vi "GlobalIniInputOutput.vi"(9 "Read or Write":T1=enum."Read Key", 11 "Ini File Refnum":T2) -> ()   [LabVIEW 2014]
uses:
  <vilib>/Utility/config.llb/Config Data RefNum.ctl
  ReadWriteIniKey.ctl
  Robot Global Data.vi
  AutonCals.vi
  DriveCals.vi
  <vilib>/Utility/config.llb/NI_LVConfig.lvlib
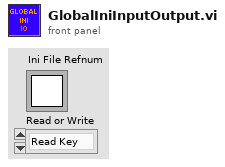
[diagram p1: front panel]
types:
  T1 = typedef "ReadWriteIniKey.ctl" = enum16{"Write Key", "Read Key"}
  T2 = typedef "NI_LVConfig.lvlib/Config Data RefNum.ctl" = refnum<k1>
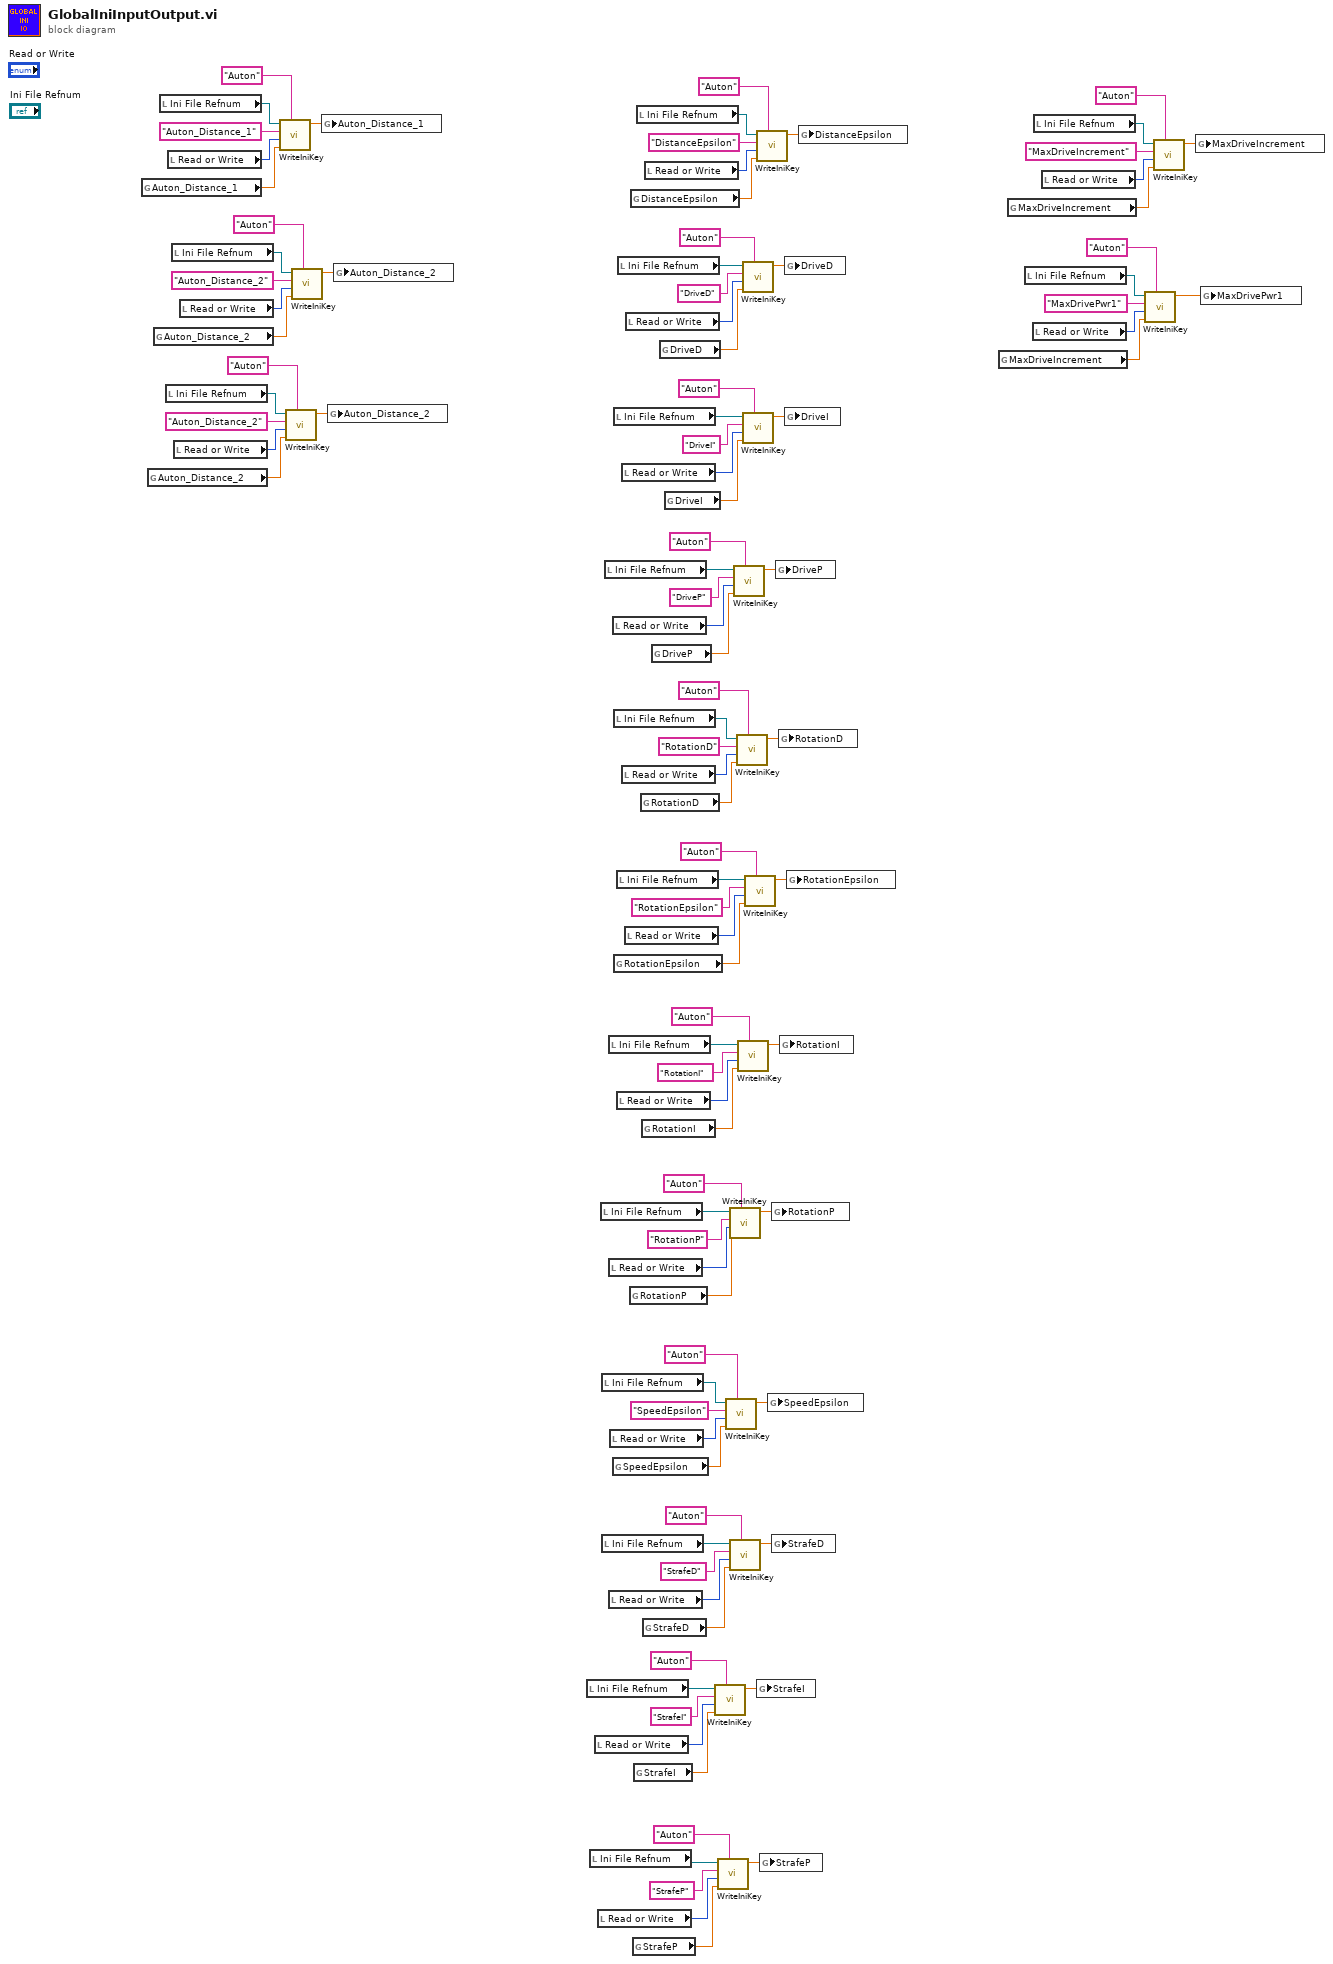
[diagram p0: block diagram]
diagram:
  n1 = global read "Robot Global Data.vi" "Auton_Distance_1"() -> (w96:dbl)
  n2 = global read "Robot Global Data.vi" "Auton_Distance_2"() -> (w90:dbl)
  n3 = global read "Robot Global Data.vi" "Auton_Distance_2"() -> (w97:dbl)
  n4 = local read "Ini File Refnum"() -> (w92:T2)
  n5 = local read "Ini File Refnum"() -> (w86:T2)
  n6 = local read "Read or Write"() -> (w91:T1)
  n7 = local read "Ini File Refnum"() -> (w101:T2)
  n8 = local read "Read or Write"() -> (w85:T1)
  n9 = local read "Read or Write"() -> (w102:T1)
  n10 = call "WriteIniKey.vi"("Section Name"="Auton", "Key Val In"=w96, 9:w91, "Key Name"="Auton_Distance_1", "Ini File Refnum"=w92) -> ("Key Val Out"=w95:dbl)  [unwired: 6 in]
  n11 = call "WriteIniKey.vi"("Section Name"="Auton", "Key Val In"=w90, 9:w85, "Key Name"="Auton_Distance_2", "Ini File Refnum"=w86) -> ("Key Val Out"=w89:dbl)  [unwired: 6 in]
  n12 = call "WriteIniKey.vi"("Section Name"="Auton", "Key Val In"=w97, 9:w102, "Key Name"="Auton_Distance_2", "Ini File Refnum"=w101) -> ("Key Val Out"=w98:dbl)  [unwired: 6 in]
  n13 = global write "Robot Global Data.vi" "Auton_Distance_1"(w95) -> ()
  n14 = global write "Robot Global Data.vi" "Auton_Distance_2"(w89) -> ()
  n15 = global write "Robot Global Data.vi" "Auton_Distance_2"(w98) -> ()
  n16 = local read "Ini File Refnum"() -> (w33:T2)
  n17 = local read "Ini File Refnum"() -> (w26:T2)
  n18 = local read "Read or Write"() -> (w34:T1)
  n19 = local read "Read or Write"() -> (w25:T1)
  n20 = local read "Ini File Refnum"() -> (w46:T2)
  n21 = local read "Ini File Refnum"() -> (w43:T2)
  n22 = local read "Ini File Refnum"() -> (w36:T2)
  n23 = local read "Ini File Refnum"() -> (w66:T2)
  n24 = local read "Ini File Refnum"() -> (w53:T2)
  n25 = local read "Read or Write"() -> (w45:T1)
  n26 = local read "Read or Write"() -> (w35:T1)
  n27 = local read "Read or Write"() -> (w44:T1)
  n28 = local read "Read or Write"() -> (w65:T1)
  n29 = global read "AutonCals.vi" "SpeedEpsilon"() -> (w20:dbl)
  n30 = local read "Ini File Refnum"() -> (w73:T2)
  n31 = local read "Ini File Refnum"() -> (w63:T2)
  n32 = global read "AutonCals.vi" "RotationEpsilon"() -> (w17:dbl)
  n33 = local read "Ini File Refnum"() -> (w56:T2)
  n34 = local read "Read or Write"() -> (w54:T1)
  n35 = local read "Ini File Refnum"() -> (w76:T2)
  n36 = local read "Read or Write"() -> (w74:T1)
  n37 = local read "Read or Write"() -> (w64:T1)
  n38 = local read "Read or Write"() -> (w55:T1)
  n39 = local read "Read or Write"() -> (w75:T1)
  n40 = global read "AutonCals.vi" "RotationP"() -> (w19:dbl)
  n41 = global read "AutonCals.vi" "DistanceEpsilon"() -> (w24:dbl)
  n42 = global read "AutonCals.vi" "StrafeP"() -> (w23:dbl)
  n43 = global read "AutonCals.vi" "StrafeI"() -> (w22:dbl)
  n44 = local read "Ini File Refnum"() -> (w83:T2)
  n45 = global read "AutonCals.vi" "RotationD"() -> (w16:dbl)
  n46 = global read "AutonCals.vi" "RotationI"() -> (w18:dbl)
  n47 = global read "AutonCals.vi" "StrafeD"() -> (w21:dbl)
  n48 = local read "Read or Write"() -> (w84:T1)
  n49 = global read "AutonCals.vi" "DriveP"() -> (w15:dbl)
  n50 = global read "AutonCals.vi" "DriveD"() -> (w13:dbl)
  n51 = global read "AutonCals.vi" "DriveI"() -> (w14:dbl)
  n52 = call "WriteIniKey.vi"("Section Name"="Auton", "Key Val In"=w22, 9:w34, "Key Name"="StrafeI", "Ini File Refnum"=w33) -> ("Key Val Out"=w30:dbl)  [unwired: 6 in]
  n53 = call "WriteIniKey.vi"("Section Name"="Auton", "Key Val In"=w23, 9:w25, "Key Name"="StrafeP", "Ini File Refnum"=w26) -> ("Key Val Out"=w29:dbl)  [unwired: 6 in]
  n54 = call "WriteIniKey.vi"("Section Name"="Auton", "Key Val In"=w20, 9:w44, "Key Name"="SpeedEpsilon", "Ini File Refnum"=w43) -> ("Key Val Out"=w40:dbl)  [unwired: 6 in]
  n55 = call "WriteIniKey.vi"("Section Name"="Auton", "Key Val In"=w19, 9:w45, "Key Name"="RotationP", "Ini File Refnum"=w46) -> ("Key Val Out"=w49:dbl)  [unwired: 6 in]
  n56 = call "WriteIniKey.vi"("Section Name"="Auton", "Key Val In"=w21, 9:w35, "Key Name"="StrafeD", "Ini File Refnum"=w36) -> ("Key Val Out"=w39:dbl)  [unwired: 6 in]
  n57 = call "WriteIniKey.vi"("Section Name"="Auton", "Key Val In"=w15, 9:w65, "Key Name"="DriveP", "Ini File Refnum"=w66) -> ("Key Val Out"=w69:dbl)  [unwired: 6 in]
  n58 = call "WriteIniKey.vi"("Section Name"="Auton", "Key Val In"=w16, 9:w64, "Key Name"="RotationD", "Ini File Refnum"=w63) -> ("Key Val Out"=w60:dbl)  [unwired: 6 in]
  n59 = call "WriteIniKey.vi"("Section Name"="Auton", "Key Val In"=w18, 9:w54, "Key Name"="RotationI", "Ini File Refnum"=w53) -> ("Key Val Out"=w50:dbl)  [unwired: 6 in]
  n60 = call "WriteIniKey.vi"("Section Name"="Auton", "Key Val In"=w13, 9:w75, "Key Name"="DriveD", "Ini File Refnum"=w76) -> ("Key Val Out"=w79:dbl)  [unwired: 6 in]
  n61 = call "WriteIniKey.vi"("Section Name"="Auton", "Key Val In"=w14, 9:w74, "Key Name"="DriveI", "Ini File Refnum"=w73) -> ("Key Val Out"=w70:dbl)  [unwired: 6 in]
  n62 = call "WriteIniKey.vi"("Section Name"="Auton", "Key Val In"=w17, 9:w55, "Key Name"="RotationEpsilon", "Ini File Refnum"=w56) -> ("Key Val Out"=w59:dbl)  [unwired: 6 in]
  n63 = call "WriteIniKey.vi"("Section Name"="Auton", "Key Val In"=w24, 9:w84, "Key Name"="DistanceEpsilon", "Ini File Refnum"=w83) -> ("Key Val Out"=w80:dbl)  [unwired: 6 in]
  n64 = global write "AutonCals.vi" "StrafeI"(w30) -> ()
  n65 = global write "AutonCals.vi" "StrafeP"(w29) -> ()
  n66 = global write "AutonCals.vi" "SpeedEpsilon"(w40) -> ()
  n67 = global write "AutonCals.vi" "RotationP"(w49) -> ()
  n68 = global write "AutonCals.vi" "StrafeD"(w39) -> ()
  n69 = global write "AutonCals.vi" "DriveP"(w69) -> ()
  n70 = global write "AutonCals.vi" "RotationD"(w60) -> ()
  n71 = global write "AutonCals.vi" "RotationI"(w50) -> ()
  n72 = global write "AutonCals.vi" "DriveD"(w79) -> ()
  n73 = global write "AutonCals.vi" "DriveI"(w70) -> ()
  n74 = global write "AutonCals.vi" "RotationEpsilon"(w59) -> ()
  n75 = global write "AutonCals.vi" "DistanceEpsilon"(w80) -> ()
  n76 = global read "DriveCals.vi" "MaxDriveIncrement"() -> (w6:dbl)
  n77 = global read "DriveCals.vi" "MaxDriveIncrement"() -> (w7:dbl)
  n78 = local read "Ini File Refnum"() -> (w3:T2)
  n79 = local read "Read or Write"() -> (w4:T1)
  n80 = local read "Ini File Refnum"() -> (w10:T2)
  n81 = local read "Read or Write"() -> (w9:T1)
  n82 = call "WriteIniKey.vi"("Section Name"="Auton", "Key Val In"=w6, 9:w4, "Key Name"="MaxDrivePwr1", "Ini File Refnum"=w3) -> ("Key Val Out"=w5:dbl)  [unwired: 6 in]
  n83 = call "WriteIniKey.vi"("Section Name"="Auton", "Key Val In"=w7, 9:w9, "Key Name"="MaxDriveIncrement", "Ini File Refnum"=w10) -> ("Key Val Out"=w8:dbl)  [unwired: 6 in]
  n84 = global write "DriveCals.vi" "MaxDriveIncrement"(w8) -> ()
  n85 = global write "DriveCals.vi" "MaxDrivePwr1"(w5) -> ()
